vi "Seconds to Time.vi"(1 "Seconds":dbl[unit]) -> (0 "Time":string)   [LabVIEW 2009]
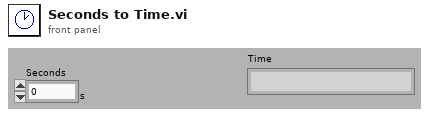
[diagram p1: front panel]
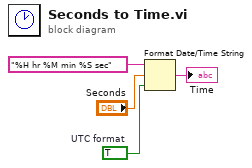
[diagram p0: block diagram]
diagram:
  w2 = TRUE  # UTC format
  n1 = Format Date/Time String(time format string (%c)="%H hr %M min %S sec", seconds (now)="Seconds", UTC format=w2) -> (date/time string=→"Time":string)
